vi "GetFolderSize.vi"(8 "Error In":errorcluster, 10 "Folder":string[](array[string]), 11 "object in":refnum<class "2022_7.lvclass">) -> (0 "Error Out":errorcluster, 2 "Size":u64, 3 "object out":refnum<class "2022_7.lvclass">)   [LabVIEW 2020, in "2022_7.lvclass"]
uses:
  2022_7.lvclass
  2022_7.lvclass/2022_7.ctl
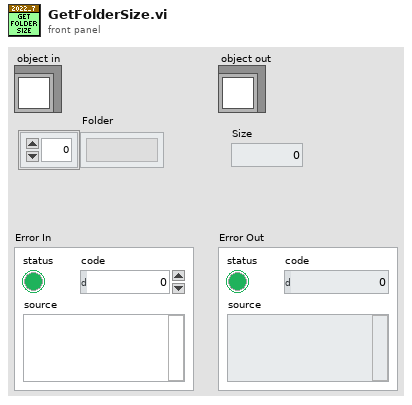
[diagram p1: front panel]
types:
  T1 = map{string[], cluster{"Folders":string[], "Files":cluster{"Name":string, "Size":i32}[]}}
  T2 = cluster{"Folders":string[], "Files":cluster{"Name":string, "Size":i32}[]}
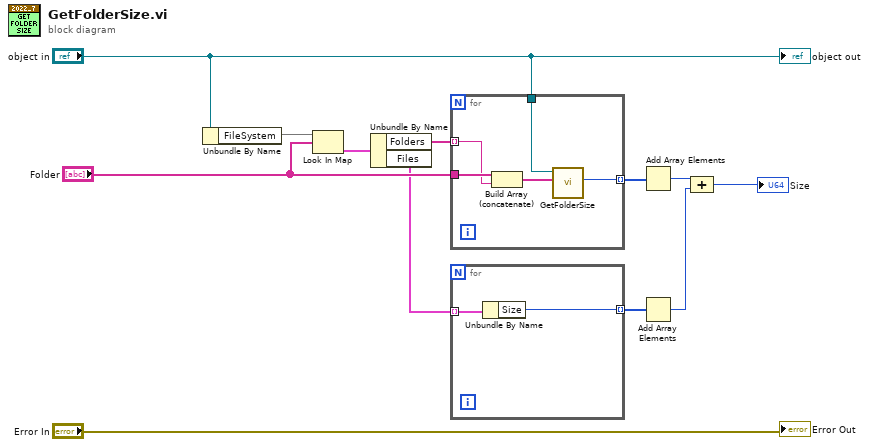
[diagram p0: block diagram]
diagram:
  n1 = Unbundle By Name("object in") -> ("FileSystem"=w11:T1)
  n2 = Look In Map(map=w11, key="Folder") -> (value=w10:T2)  [unwired: 1 in, 1 out]
  n3 = Unbundle By Name(w10) -> ("Folders"=w8:string[], "Files"=w5:cluster{"Name":string, "Size":i32}[])
  n4 = for {
    tunnel: "Folder" -> [w17]
    tunnel: w8 -> [w16] mode=indexing
    tunnel: "object in" -> [w14]
    tunnel: [w13] -> w4 mode=indexing
    n5 = Build Array (concatenate)(w17, w16) -> (w15:string[])
    n6 = call "GetFolderSize.vi"("Folder"=w15, "object in"=w14) -> ("Size"=w13:u64)  [unwired: 7 in, 2 out]
  }
  n7 = for {
    tunnel: w5 -> [w19] mode=indexing
    tunnel: [w18] -> w2 mode=indexing
    n8 = Unbundle By Name(w19) -> ("Size"=w18:i32)
  }
  n9 = Add Array Elements(numeric array=w4) -> (sum=w3:u64)
  n10 = Add Array Elements(numeric array=w2) -> (sum=w1:i32)
  n11 = Compound Arithmetic op=ADD(w3, w1) -> (→"Size":u64)
  "Error Out" <- "Error In"
  "object out" <- "object in"
